vi "Split WAVEFORM array in half.vi"(8 "error in (no error)":errorcluster, 10 "AO Array":waveform(dbl)[](array[waveform])) -> (0 "error out":errorcluster, 2 "Array 2":waveform(dbl)[](array[waveform]), 3 "Array 1":waveform(dbl)[](array[waveform]))   [LabVIEW 2020, in "DSP_lockin.lvclass"]
uses:
  DSP_lockin.lvclass
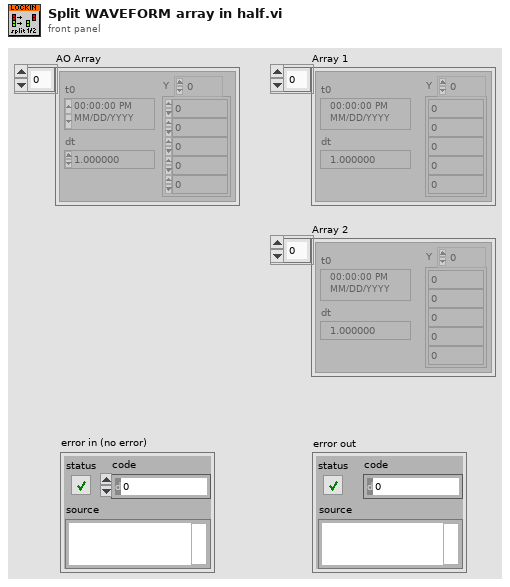
[diagram p1: front panel]
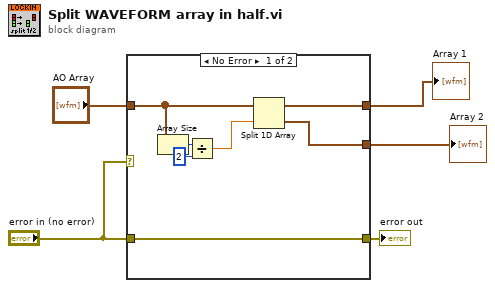
[diagram p0: block diagram]
diagram:
  n1 = case shown="No Error" "error in (no error)" {
    tunnel: [w10 _] -> w5
    tunnel: [w9 _] -> w4
    tunnel: "AO Array" -> [w8 _]
    tunnel: [w6 w13] -> w1
    tunnel: "error in (no error)" -> [w6 w13]
    frame No Error {
      n2 = Array Size(array=w8) -> (size(s)=w11:i32)
      n3 = Divide(x=w11, y=2) -> (x/y=w7:dbl)
      n4 = Split 1D Array(array=w8, index=w7) -> (first subarray=w9:waveform(dbl)[], second subarray=w10:waveform(dbl)[])
    }
    frame Error {
    }
  }
  "Array 2" <- w5
  "Array 1" <- w4
  "error out" <- w1
